vi "EasyDAQ.vi"() -> ()   [LabVIEW 2011]
panel:
  out "Offsets":dbl[](array[numeric])
  out "Gains":dbl[](array[numeric])
  out "Gain 5":i32
  out "P-Channel":i32
  out "NumBytes":i32
  out "N-channel":i32
  out "NumChannel":i32
  out "DATA":dbl
  in  "Quit":bool
  out "connected to device":bool
  in  "VISA resource Input":refnum<visa-resource-name>
  in  "Boolean 3":bool
  in  "Boolean 2":bool
  in  "Boolean 1":bool
  in  "Boolean":bool
  out "Waveform Graph":waveform(dbl)(graph)
  in  "Rate (ms) 3":dbl=500.0
  in  "Rate (ms) 2":dbl=500.0
  in  "Rate (ms) 2":dbl=500.0
  in  "Rate (ms)":dbl=500.0
  out "Final Value 4":dbl
  in  "Offset 4":dbl
  in  "Gain 4":dbl
  out "Voltage 4":dbl
  in  "Name 4":string
  in  "Range  4":string(combo)="1"
  in  "Ch-  4":string(combo)="0"
  in  "Ch+ 4":string(combo)="4"
  out "Final Value 3":dbl
  in  "Offset 3":dbl
  in  "Gain 3":dbl
  out "Voltage 3":dbl
  in  "Name 3":string
  in  "Range  3":string(combo)="1"
  in  "Ch-  3":string(combo)="0"
  in  "Ch+ 3":string(combo)="5"
  out "Final Value 2":dbl
  in  "Offset 2":dbl
  in  "Gain 2":dbl
  out "Voltage 2":dbl
  in  "Name 2":string
  in  "Range  2":string(combo)="1"
  in  "Ch-  2":string(combo)="0"
  in  "Ch+ 2":string(combo)="6"
  out "Final Value":dbl
  in  "Offset":dbl
  in  "Gain":dbl
  out "Voltage":dbl
  in  "Name":string
  in  "OK Button":bool
  in  "?":bool
  in  "Range":string(combo)="1"
  in  "Ch-":string(combo)="0"
  in  "Ch+":string(combo)="7"
  # "Experiment 1:"
  # "Experiment 2:"
  # "Experiment 3:"
  # "Experiment 4:"
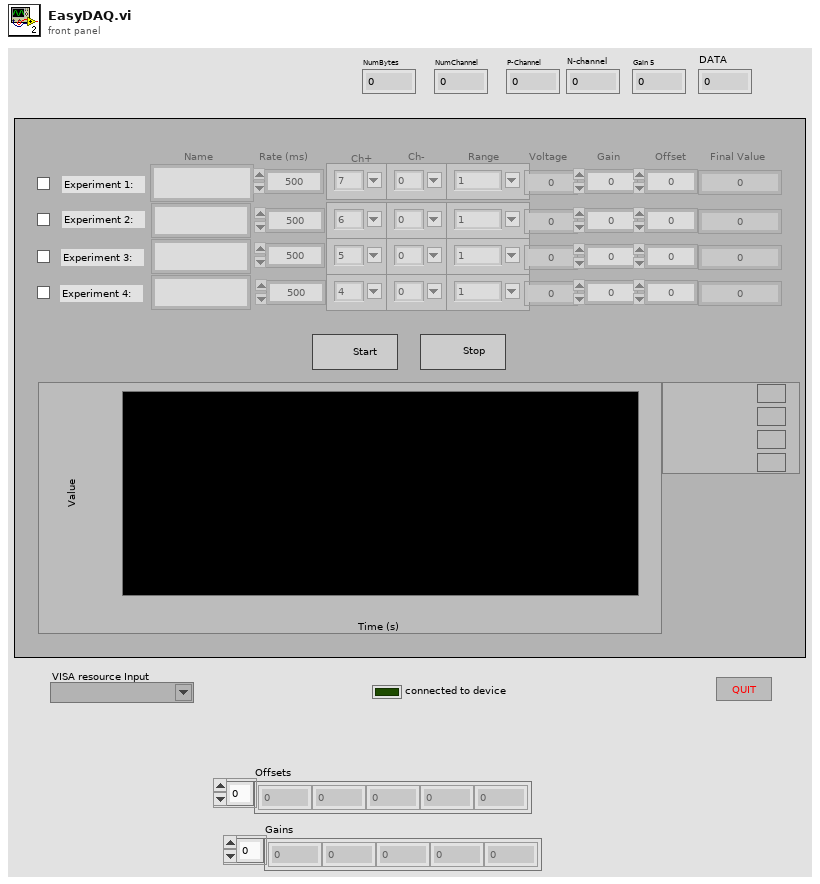
[diagram p1: front panel]
types:
  T1 = enum8{"Enabled", "Disabled", "Disabled and Grayed Out"}
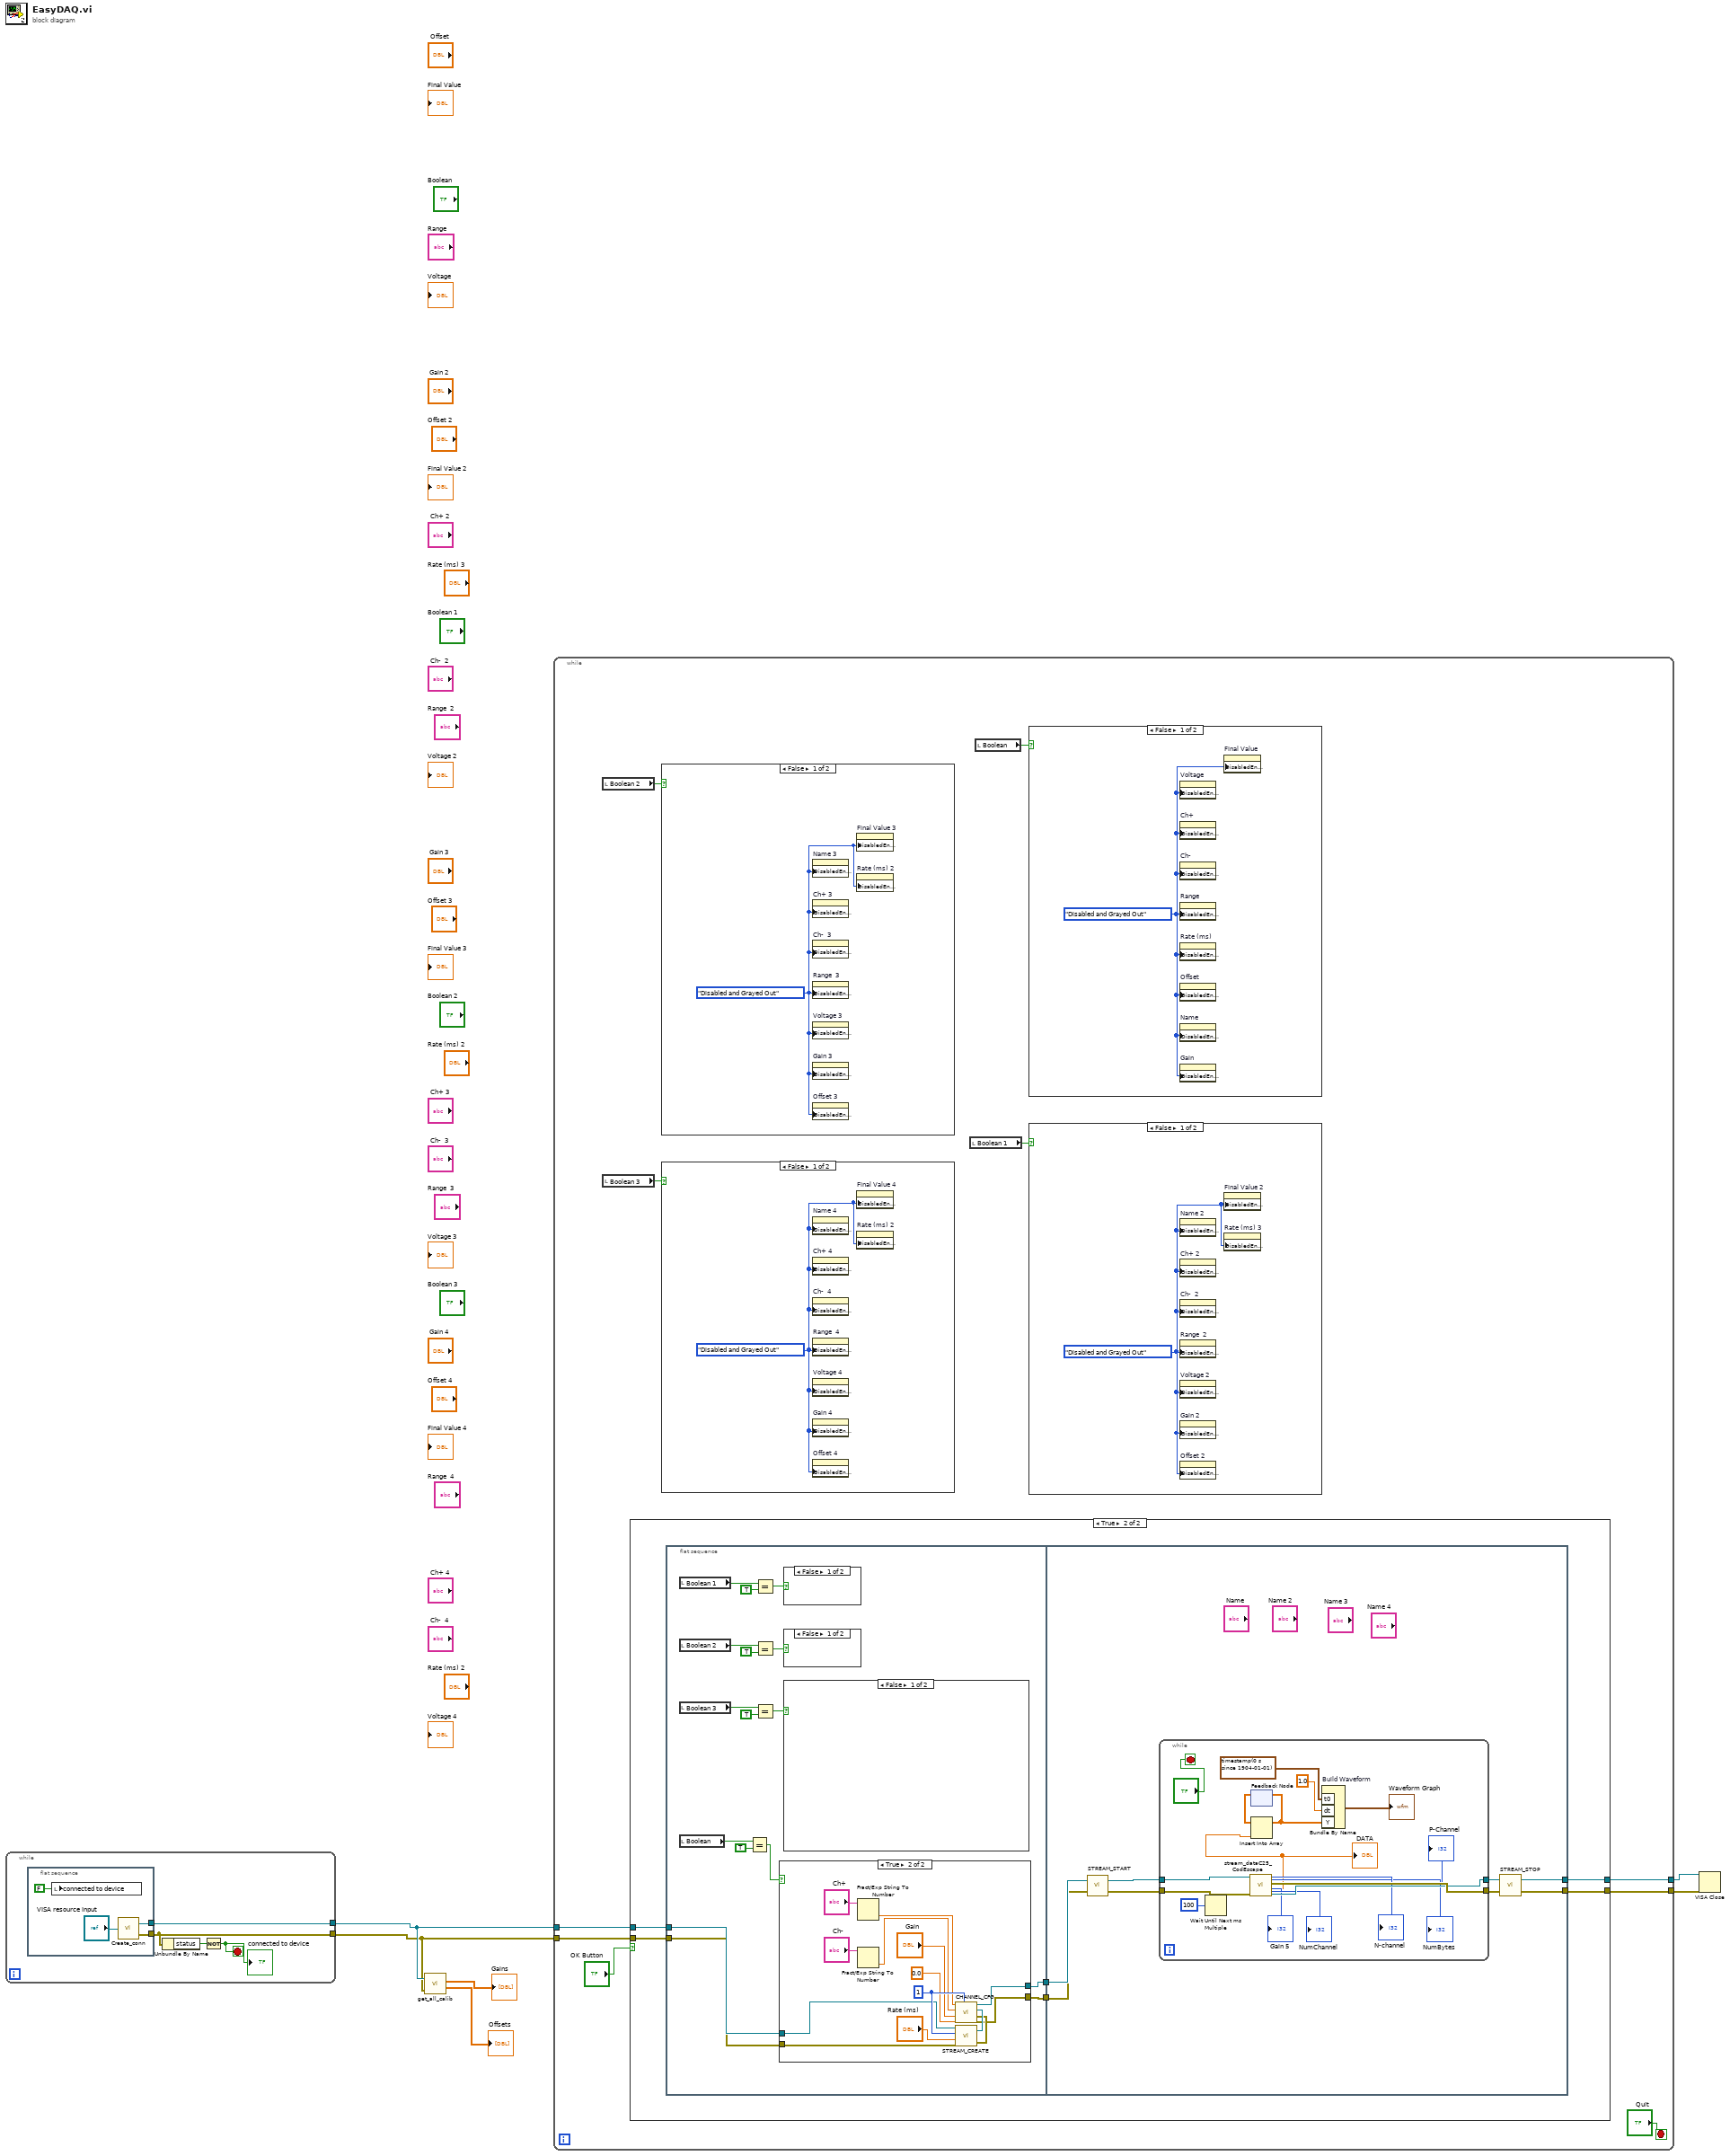
[diagram p0: block diagram]
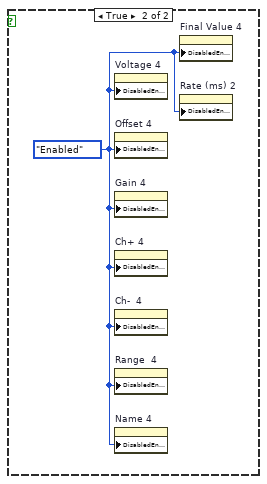
[diagram p2: hidden frame]
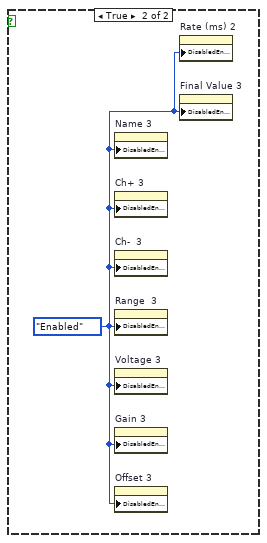
[diagram p3: hidden frame]
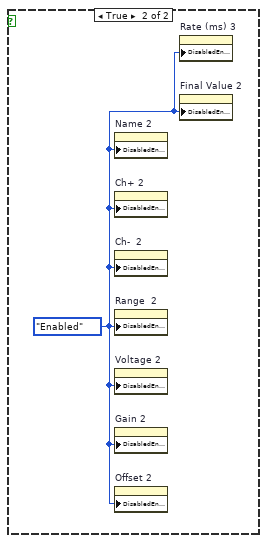
[diagram p4: hidden frame]
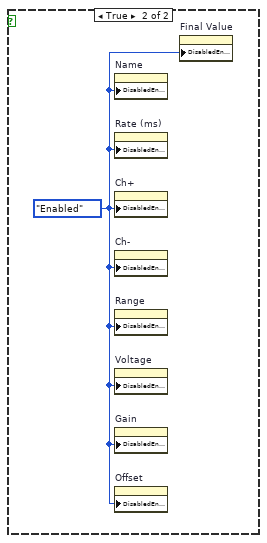
[diagram p5: hidden frame]
diagram:
  n1 = while {
    tunnel: [w10] -> w2
    tunnel: [w9] -> w1
    stop <- w7 stop-if-true
    n2 = flat-sequence {
      tunnel: [w14] -> w10
      tunnel: [w13] -> w9
      frame #0 {
        n3 = local write "connected to device"(FALSE ("connected to device")) -> ()
        n4 = call "Create_conn.vi"("VISA resourceINPUT"="VISA resource Input") -> ("error out"=w13:errorcluster, "VISA resource name out"=w14:refnum<visa-resource-name>)
      }
    }
    n5 = Unbundle By Name(w9) -> ("status"=w8:bool)
    n6 = Not(x=w8) -> (.not. x?=w7:bool)
    "connected to device" <- w7
  }
  n7 = call "get_all_calib.vi"("VISA resource name"=w2, "error in (no error)"=w1) -> ("Gains"=→"Gains":dbl[], "Offsets"=→"Offsets":dbl[])  [unwired: 2 out]
  n8 = while {
    tunnel: w2 -> [w23]
    tunnel: w1 -> [w22]
    tunnel: [w16] -> w6
    tunnel: [w15] -> w5
    stop <- "Quit" stop-if-true
    n9 = local read "Boolean 2"() -> (w19:bool)
    n10 = local read "Boolean 3"() -> (w18:bool)
    n11 = case shown="True" "OK Button" {
      tunnel: w23 -> [_ w36]
      tunnel: w22 -> [_ w35]
      tunnel: [_ w34] -> w16
      tunnel: [_ w33] -> w15
      frame False {
      }
      frame True {
        n12 = flat-sequence {
          tunnel: w36 -> [w54]
          tunnel: w35 -> [w53]
          tunnel: [w52] -> w38
          tunnel: [w51] -> w37
          tunnel: w38 -> [w74]
          tunnel: w37 -> [w73]
          tunnel: [w70] -> w34
          tunnel: [w69] -> w33
          frame #0 {
            n13 = local read "Boolean 1"() -> (w50:bool)
            n14 = local read "Boolean 2"() -> (w46:bool)
            n15 = local read "Boolean 3"() -> (w43:bool)
            n16 = local read "Boolean"() -> (w41:bool)
            n17 = Equal?(x=w41, y=TRUE) -> (x = y?=w39:bool)
            n18 = Equal?(x=w50, y=TRUE) -> (x = y?=w48:bool)
            n19 = Equal?(x=w46, y=TRUE) -> (x = y?=w47:bool)
            n20 = Equal?(x=w43, y=TRUE) -> (x = y?=w44:bool)
            n21 = case shown="True" w39 {
              tunnel: [_ w58] -> w52
              tunnel: [_ w57] -> w51
              tunnel: w54 -> [_ w56]
              tunnel: w53 -> [_ w55]
              frame False {
              }
              frame True {
                w66 = i8 1 ("Channel")
                n22 = Fract/Exp String To Number(string="Ch+") -> (number=w61:dbl)  [unwired: 3 in, 1 out]
                n23 = Fract/Exp String To Number(string="Ch-") -> (number=w59:dbl)  [unwired: 3 in, 1 out]
                n24 = call "STREAM_CREATE.vi"("error in (no error)"=w55, "Period"="Rate (ms)", "Channel"=w66, "VISA resource Input"=w56) -> ("error out"=w64:errorcluster, "VISA resource name out"=w67:refnum<visa-resource-name>)
                n25 = call "CHANNEL_CFG.vi"("error in (no error)"=w64, "VISA resource name"=w67, "Channel"=w66, "Mode"=0.0, "Gain"="Gain", "Nchan"=w59, "Pchan"=w61) -> ("error out"=w57:errorcluster, "VISA resource name out"=w58:refnum<visa-resource-name>)
              }
            }
            n26 = case shown="False" w48 {
              frame False {
              }
              frame True {
              }
            }
            n27 = case shown="False" w47 {
              frame False {
              }
              frame True {
              }
            }
            n28 = case shown="False" w44 {
              frame False {
              }
              frame True {
              }
            }
          }
          frame #1 {
            n29 = call "STREAM_START.vi"("error in (no error)"=w73, "VISA resource Input"=w74) -> ("error out"=w76:errorcluster, "VISA resource name out"=w75:refnum<visa-resource-name>)
            n30 = while {
              tunnel: w75 -> [w87]
              tunnel: w76 -> [w86]
              tunnel: [w84] -> w72
              tunnel: [w85] -> w71
              stop <- "?" stop-if-true
              n31 = Wait Until Next ms Multiple(millisecond multiple=u32 100) -> ()  [unwired: 1 out]
              n32 = call "stream_dataC25_CodEscape.vi"("VISA resource name out 2"=w87, "error out 2"=w86) -> ("error out"=w85:errorcluster, "Gain"=→"Gain 5":i32, "NumBytes"=→"NumBytes":i32, "NumChannel"=→"NumChannel":i32, "N-channel"=→"N-channel":i32, "P-Channel"=→"P-Channel":i32, "DATA"=w77:dbl, "VISA resource name out"=w84:refnum<visa-resource-name>)
              "DATA" <- w77
              n33 = feedback #1() -> (w93:dbl[])  [unwired: 1 in]
              n34 = Insert Into Array(array=w93, new element=w77) -> (w92:dbl[])  [unwired: 1 in]
              n35 = feedback-in #1(w92) -> ()
              n36 = Bundle By Name "Build Waveform"("t0"=timestamp(0 s since 1904-01-01), "dt"=1.0, "Y"=w92) -> (→"Waveform Graph":waveform(dbl))  [unwired: 1 in]
            }
            n37 = call "STREAM_STOP.vi"("error in (no error)"=w71, "VISA resource Input"=w72) -> ("error out"=w69:errorcluster, "VISA resource name out"=w70:refnum<visa-resource-name>)
          }
        }
      }
    }
    n38 = case shown="False" w19 {
      frame False {
        w27 = T1."Disabled and Grayed Out" ("Disabled")
        n39 = property on="Name 3" class="Str"("DisabledEnum"=w27) -> ()  [unwired: 2 in, 2 out]
        n40 = property on="Ch+ 3" class="CmbBox"("DisabledEnum"=w27) -> ()  [unwired: 2 in, 2 out]
        n41 = property on="Ch-  3" class="CmbBox"("DisabledEnum"=w27) -> ()  [unwired: 2 in, 2 out]
        n42 = property on="Range  3" class="CmbBox"("DisabledEnum"=w27) -> ()  [unwired: 2 in, 2 out]
        n43 = property on="Voltage 3" class="DigNum (strict)"("DisabledEnum"=w27) -> ()  [unwired: 2 in, 2 out]
        n44 = property on="Gain 3" class="DigNum (strict)"("DisabledEnum"=w27) -> ()  [unwired: 2 in, 2 out]
        n45 = property on="Offset 3" class="DigNum (strict)"("DisabledEnum"=w27) -> ()  [unwired: 2 in, 2 out]
        n46 = property on="Final Value 3" class="DigNum (strict)"("DisabledEnum"=w27) -> ()  [unwired: 2 in, 2 out]
        n47 = property on="Rate (ms) 2" class="DigNum (strict)"("DisabledEnum"=w27) -> ()  [unwired: 2 in, 2 out]
      }
      frame True {
        w28 = T1."Enabled" ("Disabled")
        n48 = property on="Name 3" class="Str"("DisabledEnum"=w28) -> ()  [unwired: 2 in, 2 out]
        n49 = property on="Ch+ 3" class="CmbBox"("DisabledEnum"=w28) -> ()  [unwired: 2 in, 2 out]
        n50 = property on="Ch-  3" class="CmbBox"("DisabledEnum"=w28) -> ()  [unwired: 2 in, 2 out]
        n51 = property on="Range  3" class="CmbBox"("DisabledEnum"=w28) -> ()  [unwired: 2 in, 2 out]
        n52 = property on="Voltage 3" class="DigNum (strict)"("DisabledEnum"=w28) -> ()  [unwired: 2 in, 2 out]
        n53 = property on="Gain 3" class="DigNum (strict)"("DisabledEnum"=w28) -> ()  [unwired: 2 in, 2 out]
        n54 = property on="Offset 3" class="DigNum (strict)"("DisabledEnum"=w28) -> ()  [unwired: 2 in, 2 out]
        n55 = property on="Rate (ms) 2" class="DigNum (strict)"("DisabledEnum"=w28) -> ()  [unwired: 2 in, 2 out]
        n56 = property on="Final Value 3" class="DigNum (strict)"("DisabledEnum"=w28) -> ()  [unwired: 2 in, 2 out]
      }
    }
    n57 = case shown="False" w18 {
      frame False {
        w25 = T1."Disabled and Grayed Out" ("Disabled")
        n58 = property on="Name 4" class="Str"("DisabledEnum"=w25) -> ()  [unwired: 2 in, 2 out]
        n59 = property on="Ch+ 4" class="CmbBox"("DisabledEnum"=w25) -> ()  [unwired: 2 in, 2 out]
        n60 = property on="Ch-  4" class="CmbBox"("DisabledEnum"=w25) -> ()  [unwired: 2 in, 2 out]
        n61 = property on="Range  4" class="CmbBox"("DisabledEnum"=w25) -> ()  [unwired: 2 in, 2 out]
        n62 = property on="Voltage 4" class="DigNum (strict)"("DisabledEnum"=w25) -> ()  [unwired: 2 in, 2 out]
        n63 = property on="Gain 4" class="DigNum (strict)"("DisabledEnum"=w25) -> ()  [unwired: 2 in, 2 out]
        n64 = property on="Offset 4" class="DigNum (strict)"("DisabledEnum"=w25) -> ()  [unwired: 2 in, 2 out]
        n65 = property on="Final Value 4" class="DigNum (strict)"("DisabledEnum"=w25) -> ()  [unwired: 2 in, 2 out]
        n66 = property on="Rate (ms) 2" class="DigNum (strict)"("DisabledEnum"=w25) -> ()  [unwired: 2 in, 2 out]
      }
      frame True {
        w26 = T1."Enabled" ("Disabled")
        n67 = property on="Voltage 4" class="DigNum (strict)"("DisabledEnum"=w26) -> ()  [unwired: 2 in, 2 out]
        n68 = property on="Offset 4" class="DigNum (strict)"("DisabledEnum"=w26) -> ()  [unwired: 2 in, 2 out]
        n69 = property on="Gain 4" class="DigNum (strict)"("DisabledEnum"=w26) -> ()  [unwired: 2 in, 2 out]
        n70 = property on="Ch+ 4" class="CmbBox"("DisabledEnum"=w26) -> ()  [unwired: 2 in, 2 out]
        n71 = property on="Ch-  4" class="CmbBox"("DisabledEnum"=w26) -> ()  [unwired: 2 in, 2 out]
        n72 = property on="Range  4" class="CmbBox"("DisabledEnum"=w26) -> ()  [unwired: 2 in, 2 out]
        n73 = property on="Name 4" class="Str"("DisabledEnum"=w26) -> ()  [unwired: 2 in, 2 out]
        n74 = property on="Final Value 4" class="DigNum (strict)"("DisabledEnum"=w26) -> ()  [unwired: 2 in, 2 out]
        n75 = property on="Rate (ms) 2" class="DigNum (strict)"("DisabledEnum"=w26) -> ()  [unwired: 2 in, 2 out]
      }
    }
    n76 = local read "Boolean 1"() -> (w20:bool)
    n77 = local read "Boolean"() -> (w21:bool)
    n78 = case shown="False" w21 {
      frame False {
        w31 = T1."Disabled and Grayed Out" ("Disabled")
        n79 = property on="Voltage" class="DigNum (strict)"("DisabledEnum"=w31) -> ()  [unwired: 2 in, 2 out]
        n80 = property on="Ch+" class="CmbBox"("DisabledEnum"=w31) -> ()  [unwired: 2 in, 2 out]
        n81 = property on="Ch-" class="CmbBox"("DisabledEnum"=w31) -> ()  [unwired: 2 in, 2 out]
        n82 = property on="Range" class="CmbBox"("DisabledEnum"=w31) -> ()  [unwired: 2 in, 2 out]
        n83 = property on="Rate (ms)" class="DigNum (strict)"("DisabledEnum"=w31) -> ()  [unwired: 2 in, 2 out]
        n84 = property on="Offset" class="DigNum (strict)"("DisabledEnum"=w31) -> ()  [unwired: 2 in, 2 out]
        n85 = property on="Name" class="Str"("DisabledEnum"=w31) -> ()  [unwired: 2 in, 2 out]
        n86 = property on="Gain" class="DigNum (strict)"("DisabledEnum"=w31) -> ()  [unwired: 2 in, 2 out]
        n87 = property on="Final Value" class="DigNum (strict)"("DisabledEnum"=w31) -> ()  [unwired: 2 in, 2 out]
      }
      frame True {
        w32 = T1."Enabled" ("Disabled")
        n88 = property on="Name" class="Str"("DisabledEnum"=w32) -> ()  [unwired: 2 in, 2 out]
        n89 = property on="Rate (ms)" class="DigNum (strict)"("DisabledEnum"=w32) -> ()  [unwired: 2 in, 2 out]
        n90 = property on="Ch+" class="CmbBox"("DisabledEnum"=w32) -> ()  [unwired: 2 in, 2 out]
        n91 = property on="Ch-" class="CmbBox"("DisabledEnum"=w32) -> ()  [unwired: 2 in, 2 out]
        n92 = property on="Range" class="CmbBox"("DisabledEnum"=w32) -> ()  [unwired: 2 in, 2 out]
        n93 = property on="Voltage" class="DigNum (strict)"("DisabledEnum"=w32) -> ()  [unwired: 2 in, 2 out]
        n94 = property on="Gain" class="DigNum (strict)"("DisabledEnum"=w32) -> ()  [unwired: 2 in, 2 out]
        n95 = property on="Offset" class="DigNum (strict)"("DisabledEnum"=w32) -> ()  [unwired: 2 in, 2 out]
        n96 = property on="Final Value" class="DigNum (strict)"("DisabledEnum"=w32) -> ()  [unwired: 2 in, 2 out]
      }
    }
    n97 = case shown="False" w20 {
      frame False {
        w29 = T1."Disabled and Grayed Out" ("Disabled")
        n98 = property on="Name 2" class="Str"("DisabledEnum"=w29) -> ()  [unwired: 2 in, 2 out]
        n99 = property on="Ch+ 2" class="CmbBox"("DisabledEnum"=w29) -> ()  [unwired: 2 in, 2 out]
        n100 = property on="Ch-  2" class="CmbBox"("DisabledEnum"=w29) -> ()  [unwired: 2 in, 2 out]
        n101 = property on="Range  2" class="CmbBox"("DisabledEnum"=w29) -> ()  [unwired: 2 in, 2 out]
        n102 = property on="Voltage 2" class="DigNum (strict)"("DisabledEnum"=w29) -> ()  [unwired: 2 in, 2 out]
        n103 = property on="Gain 2" class="DigNum (strict)"("DisabledEnum"=w29) -> ()  [unwired: 2 in, 2 out]
        n104 = property on="Offset 2" class="DigNum (strict)"("DisabledEnum"=w29) -> ()  [unwired: 2 in, 2 out]
        n105 = property on="Final Value 2" class="DigNum (strict)"("DisabledEnum"=w29) -> ()  [unwired: 2 in, 2 out]
        n106 = property on="Rate (ms) 3" class="DigNum (strict)"("DisabledEnum"=w29) -> ()  [unwired: 2 in, 2 out]
      }
      frame True {
        w30 = T1."Enabled" ("Disabled")
        n107 = property on="Name 2" class="Str"("DisabledEnum"=w30) -> ()  [unwired: 2 in, 2 out]
        n108 = property on="Ch+ 2" class="CmbBox"("DisabledEnum"=w30) -> ()  [unwired: 2 in, 2 out]
        n109 = property on="Ch-  2" class="CmbBox"("DisabledEnum"=w30) -> ()  [unwired: 2 in, 2 out]
        n110 = property on="Range  2" class="CmbBox"("DisabledEnum"=w30) -> ()  [unwired: 2 in, 2 out]
        n111 = property on="Voltage 2" class="DigNum (strict)"("DisabledEnum"=w30) -> ()  [unwired: 2 in, 2 out]
        n112 = property on="Gain 2" class="DigNum (strict)"("DisabledEnum"=w30) -> ()  [unwired: 2 in, 2 out]
        n113 = property on="Offset 2" class="DigNum (strict)"("DisabledEnum"=w30) -> ()  [unwired: 2 in, 2 out]
        n114 = property on="Rate (ms) 3" class="DigNum (strict)"("DisabledEnum"=w30) -> ()  [unwired: 2 in, 2 out]
        n115 = property on="Final Value 2" class="DigNum (strict)"("DisabledEnum"=w30) -> ()  [unwired: 2 in, 2 out]
      }
    }
  }
  n116 = VISA Close(VISA resource name=w6, error in (no error)=w5) -> ()  [unwired: 1 out]
